vi "Radau5_Termination Criterion.vi"(7 "First call?":bool, 8 "Newton index":i32, 9 "Error TOL":dbl[](array[numeric]), 10 "Old Delta Z":dbl[](array[numeric]), 11 "Delta Z":dbl[](array[numeric])) -> (3 "Newton status":T1)   [LabVIEW 2020, in "NI_DAE.lvlib"]
uses:
  <vilib>/gmath/NI_DAE.lvlib
  <vilib>/gmath/dae.llb/Radau5_Newton Status.ctl
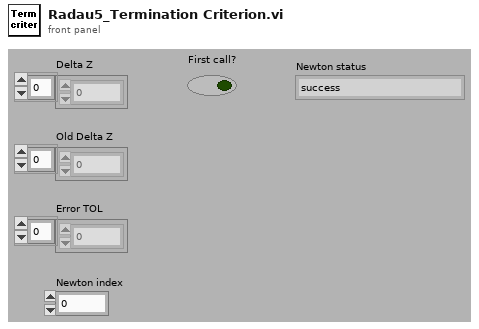
[diagram p1: front panel]
types:
  T1 = typedef "NI_DAE.lvlib/Radau5_Newton Status.ctl" = enum16{"success", "unsuccess(iteration diverge)", "unsuccess(exceed max_N)", "unsuccess(conv rate too slow)", "Continue next Newton"}
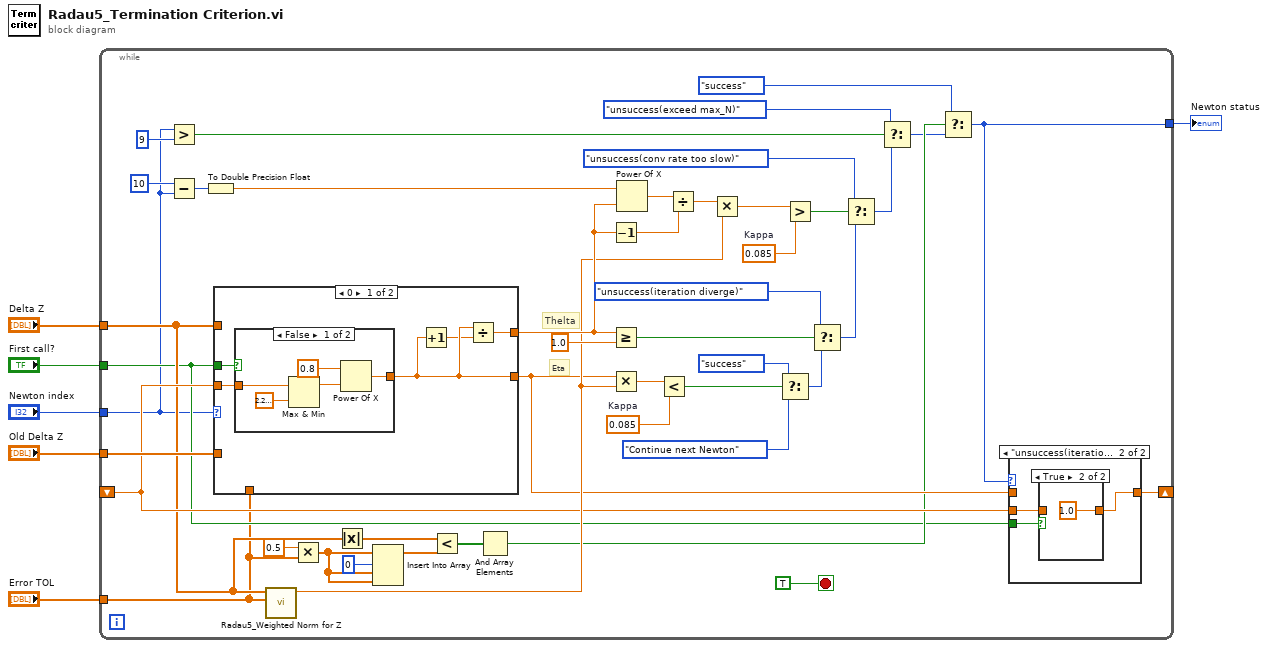
[diagram p0: block diagram]
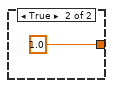
[diagram p4: hidden frame]
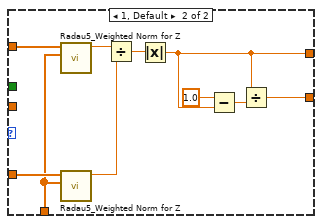
[diagram p5: hidden frame]
diagram:
  n1 = while {
    tunnel: "First call?" -> [w12]
    tunnel: "Old Delta Z" -> [w51]
    tunnel: "Delta Z" -> [w22]
    tunnel: "Error TOL" -> [w7]
    tunnel: "Newton index" -> [w11]
    tunnel: [w8] -> w1
    shift-right: [w25] -> _
    shift-left: _ -> [w24]
    stop <- TRUE ("stop") stop-if-true
    w33 = 0.085  # Kappa
    w50 = 0.085  # Kappa
    # "Thelta"
    # "Eta"
    n2 = Greater?(x=w11, y=9) -> (0:w29:bool)
    n3 = Subtract(x=10, y=w11) -> (x-y=w40:i32)
    n4 = To Double Precision Float(number=w40) -> (double precision float=w39:dbl)
    n5 = case shown="0" w11 {
      tunnel: w12 -> [w62 _]
      tunnel: [w60 w73] -> w26
      tunnel: w24 -> [w61 _]
      tunnel: w22 -> [_ w70]
      tunnel: w51 -> [_ w71]
      tunnel: [w58 w72] -> w42
      tunnel: w7 -> [_ w69]
      frame 0 {
        n6 = case shown="False" w62 {
          tunnel: [w63 1.0] -> w60
          tunnel: w61 -> [w67 _]
          frame False {
            n7 = Max & Min(x=w67, y=2.220446049250313e-16) -> (max(x,y)=w65:dbl)  [unwired: 1 out]
            n8 = Power Of X(1:w65, 2:0.8 ("y")) -> (0:w63:dbl)
          }
          frame True {
          }
        }
        n9 = Increment(x=w60) -> (x+1=w59:dbl)
        n10 = Divide(x=w60, y=w59) -> (x/y=w58:dbl)
      }
      frame 1, Default {
        n11 = call <vilib>:"Radau5_Weighted Norm for Z.vi"("Tolerance Vector"=w69, "Increment of Z"=w70) -> ("Norm of  Z"=w78:dbl)  [unwired: 9 in]
        n12 = call <vilib>:"Radau5_Weighted Norm for Z.vi"("Tolerance Vector"=w69, "Increment of Z"=w71) -> ("Norm of  Z"=w77:dbl)  [unwired: 9 in]
        n13 = Divide(x=w78, y=w77) -> (x/y=w76:dbl)
        n14 = Absolute Value(x=w76) -> (abs(x)=w72:dbl)
        n15 = Subtract(x=1.0, y=w72) -> (x-y=w74:dbl)
        n16 = Divide(x=w72, y=w74) -> (x/y=w73:dbl)
      }
    }
    n17 = call <vilib>:"Radau5_Weighted Norm for Z.vi"("Tolerance Vector"=w7, "Increment of Z"=w22) -> ("Norm of  Z"=w35:dbl)  [unwired: 9 in]
    n18 = Multiply(x=0.5, y=w7) -> (x*y=w14:dbl[])
    n19 = Absolute Value(x=w22) -> (abs(x)=w21:dbl[])
    n20 = Insert Into Array(array=w14, index=0, new element #1=w14, new element #2=w14) -> (w13:dbl[])
    n21 = Less?(x=w21, y=w13) -> (x < y?=w20:bool[])
    n22 = And Array Elements(Boolean array=w20) -> (logical AND=w17:bool)
    n23 = Decrement(x=w42) -> (x-1=w37:dbl)
    n24 = Greater Or Equal?(x=w42, y=1.0) -> (x >= y?=w45:bool)
    n25 = Multiply(x=w26, y=w35) -> (x*y=w49:dbl)
    n26 = Power Of X(1:w42, 2:w39) -> (0:w38:dbl)
    n27 = Less?(x=w49, y=w50) -> (x < y?=w18:bool)
    n28 = Divide(x=w38, y=w37) -> (x/y=w36:dbl)
    n29 = Multiply(x=w36, y=w35) -> (x*y=w34:dbl)
    n30 = Select(t=Radau5_Newton_Status."success" ("Newton status"), s=w18, f=Radau5_Newton_Status."Continue next Newton" ("Newton status")) -> (s? t:f=w44:T1)
    n31 = Greater?(x=w34, y=w33) -> (0:w32:bool)
    n32 = Select(t=Radau5_Newton_Status."unsuccess(iteration diverge)", s=w45, f=w44) -> (s? t:f=w10:T1)
    n33 = Select(t=Radau5_Newton_Status."unsuccess(conv rate too slow)", s=w32, f=w10) -> (s? t:f=w23:T1)
    n34 = Select(t=Radau5_Newton_Status."unsuccess(exceed max_N)", s=w29, f=w23) -> (s? t:f=w9:T1)
    n35 = Select(t=Radau5_Newton_Status."success" ("f"), s=w17, f=w9) -> (s? t:f=w8:T1)
    n36 = case shown="\"unsuccess(iteration diverge)\", Default" w8 {
      tunnel: w26 -> [w52 _]
      tunnel: [w52 w53] -> w25
      tunnel: w24 -> [_ w54]
      tunnel: w12 -> [_ w55]
      frame "success" {
      }
      frame "unsuccess(iteration diverge)", Default {
        n37 = case shown="True" w55 {
          tunnel: w54 -> [w56 _]
          tunnel: [w56 1.0] -> w53
          frame False {
          }
          frame True {
          }
        }
      }
    }
  }
  "Newton status" <- w1
